vi "SRV_Queue Shutdown States.vi"(8 "error in (no error)":errorcluster, 9 "In Pico":bool, 11 "Control Queue":refnum<queue>) -> (0 "error out":errorcluster, 3 "Control Queue out":refnum<queue>)   [LabVIEW 2014]
uses:
  Support/SRV_Command-Data Queue Data Type.ctl
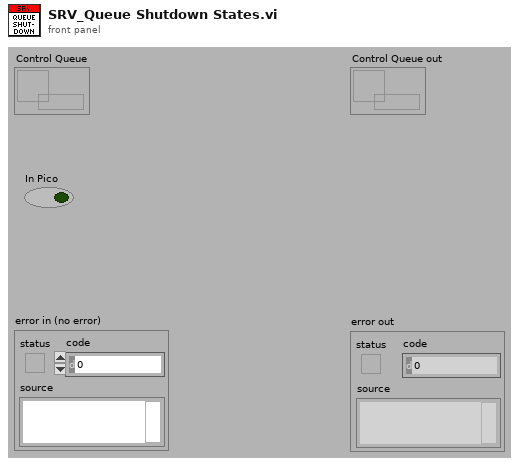
[diagram p1: front panel]
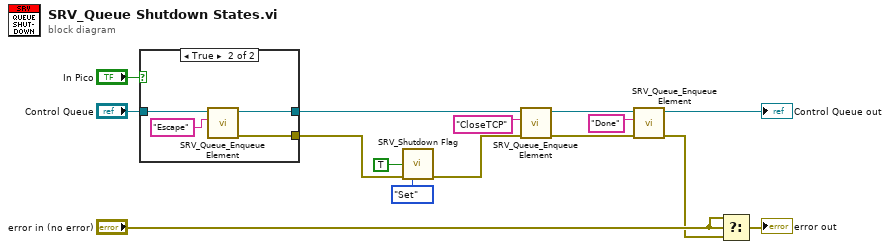
[diagram p0: block diagram]
diagram:
  n1 = case shown="True" "In Pico" {
    tunnel: "Control Queue" -> [w16 w17]
    tunnel: [w16 w19] -> w10
    tunnel: [_ w18] -> w3
    frame False {
    }
    frame True {
      n2 = call "SRV_Queue_Enqueue Element.vi"("Command"="Escape" ("name (unnamed)"), "Command-Data Queue"=w17) -> ("error out"=w18:errorcluster, "Command-Data Queue out"=w19:refnum<queue>)  [unwired: 7 in, 1 out]
    }
  }
  n3 = call "SRV_Shutdown Flag.vi"("Shutdown Flag"=TRUE ("stop"), "error in (no error)"=w3, "Method (Get)"=enum16{"Get", "Set"}."Set") -> ("error out"=w2:errorcluster)  [unwired: 11 in, 1 out]
  n4 = call "SRV_Queue_Enqueue Element.vi"("error in (no error)"=w2, "Command"="CloseTCP" ("name (unnamed)"), "Command-Data Queue"=w10) -> ("error out"=w13:errorcluster, "Command-Data Queue out"=w12:refnum<queue>)  [unwired: 6 in, 1 out]
  n5 = call "SRV_Queue_Enqueue Element.vi"("error in (no error)"=w13, "Command"="Done" ("name (unnamed)"), "Command-Data Queue"=w12) -> ("error out"=w1:errorcluster, "Command-Data Queue out"=→"Control Queue out":refnum<queue>)  [unwired: 6 in, 1 out]
  n6 = Select(t="error in (no error)", s="error in (no error)", f=w1) -> (s? t:f=→"error out":errorcluster)
